vi "MFC Setup (SubVI).vi"(0 "Refnum in":refnum<k21>, 1 "O2 MFC":string="O2", 2 "VOC MFC Channel":tag="Dev1/ai11", 3 "Scale for VOC MFC":tag="uMFC A", 4 "NOx MFC":string="NOx", 5 "error in (no error)":errorcluster, 6 "NOx MFC Channel":tag="Dev1/ai10", 7 "VOC MFC":string="VOC", 8 "N2 MFC":string="N2", 9 "Scale for N2 MFC":tag="Large MFC A", 10 "O2 MFC Channel":tag="Dev1/ai9", 11 "Scale for O2 MFC":tag="Large MFC A", 12 "N2 MFC Channel":tag="Dev1/ai8", 13 "Scale for NOx MFC":tag="uMFC A") -> (14 "Refnum out":refnum<k21>, 16 "Array":string[](array[string]), 19 "error out":errorcluster)   [LabVIEW 2011]
uses:
  <vilib>/Utility/error.llb/DialogType.ctl
  <vilib>/DAQmx/create/channels.llb/DAQmx Create Channel (AI-Voltage-Basic).vi
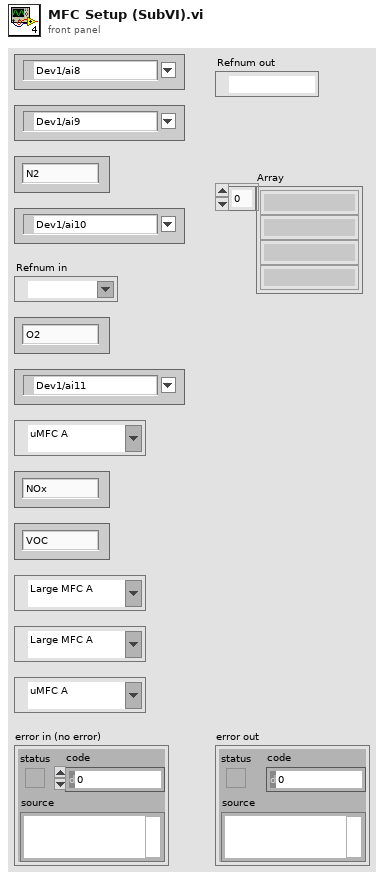
[diagram p1: front panel]
types:
  T1 = typedef "DialogType.ctl" = u16
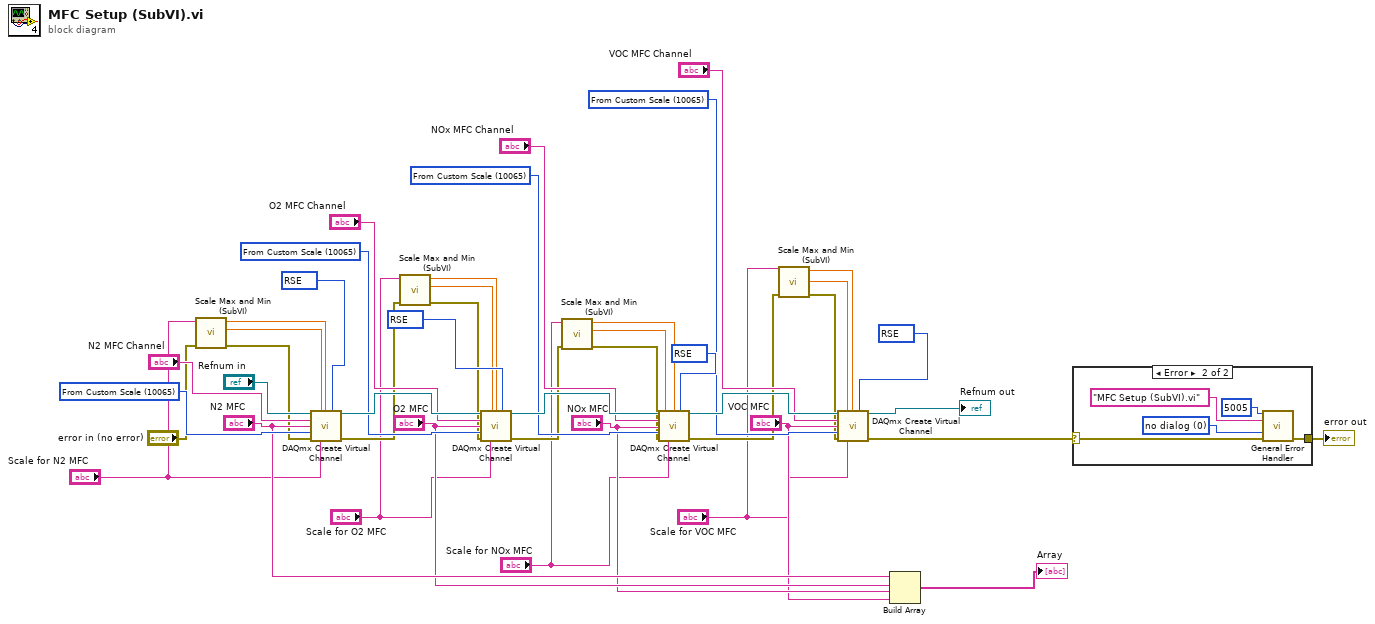
[diagram p0: block diagram]
diagram:
  w29 = 10083 items=["default"=-1, "RSE"=10083, "NRSE"=10078, "Differential"=10106, "Pseudodifferential"=12529] ("input terminal configuration")
  w30 = 10065 items=["Volts"=10348, "From Custom Scale"=10065] ("units")
  w33 = 10083 items=["default"=-1, "RSE"=10083, "NRSE"=10078, "Differential"=10106, "Pseudodifferential"=12529] ("input terminal configuration")
  w34 = 10065 items=["Volts"=10348, "From Custom Scale"=10065] ("units")
  w37 = 10083 items=["default"=-1, "RSE"=10083, "NRSE"=10078, "Differential"=10106, "Pseudodifferential"=12529] ("input terminal configuration")
  w38 = 10065 items=["Volts"=10348, "From Custom Scale"=10065] ("units")
  w42 = 10065 items=["Volts"=10348, "From Custom Scale"=10065] ("units")
  w41 = 10083 items=["default"=-1, "RSE"=10083, "NRSE"=10078, "Differential"=10106, "Pseudodifferential"=12529] ("input terminal configuration")
  n1 = call "Scale Max and Min (SubVI).vi"("error in (no error)"="error in (no error)", "Scale"="Scale for N2 MFC") -> ("error out"=w20:errorcluster, "Max"=w19:dbl, "Min"=w18:dbl)  [unwired: 7 in]
  n2 = call-poly <vilib>:"DAQmx Create Virtual Channel.vi"("task in"="Refnum in", "maximum value"=w19, "minimum value"=w18, "input terminal configuration"=w41, "physical channels"="N2 MFC Channel", "name to assign"="N2 MFC", "units"=w42, "error in"=w20, "custom scale name"="Scale for N2 MFC") -> ("task out"=w40:refnum<k21>, "error out"=w17:errorcluster)  [unwired: 5 in]
  n3 = call "Scale Max and Min (SubVI).vi"("error in (no error)"=w17, "Scale"="Scale for O2 MFC") -> ("error out"=w16:errorcluster, "Max"=w13:dbl, "Min"=w14:dbl)  [unwired: 7 in]
  n4 = call-poly <vilib>:"DAQmx Create Virtual Channel.vi"("task in"=w40, "maximum value"=w13, "minimum value"=w14, "input terminal configuration"=w37, "physical channels"="O2 MFC Channel", "name to assign"="O2 MFC", "units"=w38, "error in"=w16, "custom scale name"="Scale for O2 MFC") -> ("task out"=w36:refnum<k21>, "error out"=w12:errorcluster)  [unwired: 5 in]
  n5 = call "Scale Max and Min (SubVI).vi"("error in (no error)"=w12, "Scale"="Scale for NOx MFC") -> ("error out"=w11:errorcluster, "Max"=w8:dbl, "Min"=w9:dbl)  [unwired: 7 in]
  n6 = call-poly <vilib>:"DAQmx Create Virtual Channel.vi"("task in"=w36, "maximum value"=w8, "minimum value"=w9, "input terminal configuration"=w33, "physical channels"="NOx MFC Channel", "name to assign"="NOx MFC", "units"=w34, "error in"=w11, "custom scale name"="Scale for NOx MFC") -> ("task out"=w32:refnum<k21>, "error out"=w7:errorcluster)  [unwired: 5 in]
  n7 = call "Scale Max and Min (SubVI).vi"("error in (no error)"=w7, "Scale"="Scale for VOC MFC") -> ("error out"=w6:errorcluster, "Max"=w3:dbl, "Min"=w4:dbl)  [unwired: 7 in]
  n8 = call-poly <vilib>:"DAQmx Create Virtual Channel.vi"("task in"=w32, "maximum value"=w3, "minimum value"=w4, "input terminal configuration"=w29, "physical channels"="VOC MFC Channel", "name to assign"="VOC MFC", "units"=w30, "error in"=w6, "custom scale name"="Scale for VOC MFC") -> ("task out"=→"Refnum out":refnum<k21>, "error out"=w2:errorcluster)  [unwired: 5 in]
  n9 = Build Array("N2 MFC", "O2 MFC", "NOx MFC", "VOC MFC") -> (→"Array":string[])
  n10 = case shown="Error" w2 {
    selector: w2 -> [w45 w50]
    tunnel: [w45 w49] -> w1
    frame No Error {
    }
    frame Error {
      w47 = T1 0 items=["no dialog", "OK message", "continue or stop message", "OK message + warnings", "continue/stop + warnings"] ("type of dialog (OK msg:1)")
      n11 = call <vilib>:"General Error Handler.vi"("[error code] (0)"=5005, "[error source] (\" \")"="MFC Setup (SubVI).vi" ("[error source] (\" \")"), "type of dialog (OK msg:1)"=w47, "error in (no error)"=w50) -> ("error out"=w49:errorcluster)  [unwired: 7 in, 4 out]
    }
  }
  "error out" <- w1
